vi "ex_GetAllExpressAttribsPlus.vi"(8 "error in":errorcluster, 11 "Signals in":waveform(dbl)[](array[waveform])) -> (0 "error out":errorcluster, 1 "All Express Wave Attributes Plus":T2(array[cluster]) {"dX" format="%.2f"; "X0" format="%<%X\n%x>T"; "Timestamp" format="%<%X\n%x>T"; "Start Timestamp" format="%<%X\n%x>T"}, 2 "All Express Wave Attributes":T1(array[cluster]) {"Timestamp" format="%<%X\n%x>T"; "Start Timestamp" format="%<%X\n%x>T"}, 3 "Signals out":waveform(dbl)[](array[waveform]), 5 "Time Attribs Not Found":bool[](array[boolean]))   [LabVIEW 2020]
doc: "Read Express attributes (and other Waveform values). If any of the four time-related attributes are not found, adds a best guess to the to All Express Wave Attributes."
uses:
  ex_WaveformAttribsPlus.ctl
  ex_WaveformAttribs.ctl
panel:
  in  "origin timestamps":timestamp[](array[timestamp]) format="%<%X\n%x>T"
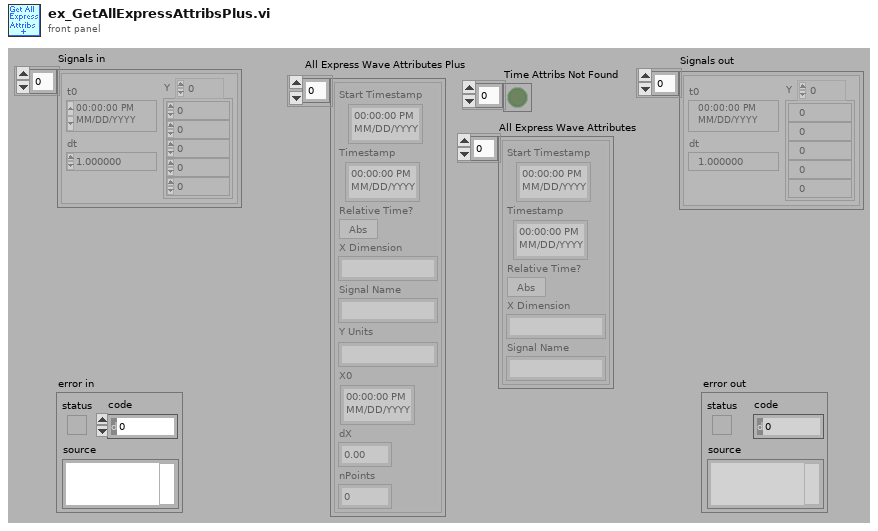
[diagram p1: front panel]
types:
  T1 = cluster{"Start Timestamp":timestamp, "Timestamp":timestamp, "Relative Time?":bool, "X Dimension":string, "Signal Name":string}[]
  T2 = cluster{"Start Timestamp":timestamp, "Timestamp":timestamp, "Relative Time?":bool, "X Dimension":string, "Signal Name":string, "Y Units":string, "X0":timestamp, "dX":dbl, "nPoints":i32}[]
  T3 = typedef "ex_WaveformAttribsPlus.ctl" = cluster{"Start Timestamp":timestamp, "Timestamp":timestamp, "Relative Time?":bool, "X Dimension":string, "Signal Name":string, "Y Units":string, "X0":timestamp, "dX":dbl, "nPoints":i32}
  T4 = typedef "ex_WaveformAttribs.ctl" = cluster{"Start Timestamp":timestamp, "Timestamp":timestamp, "Relative Time?":bool, "X Dimension":string, "Signal Name":string}
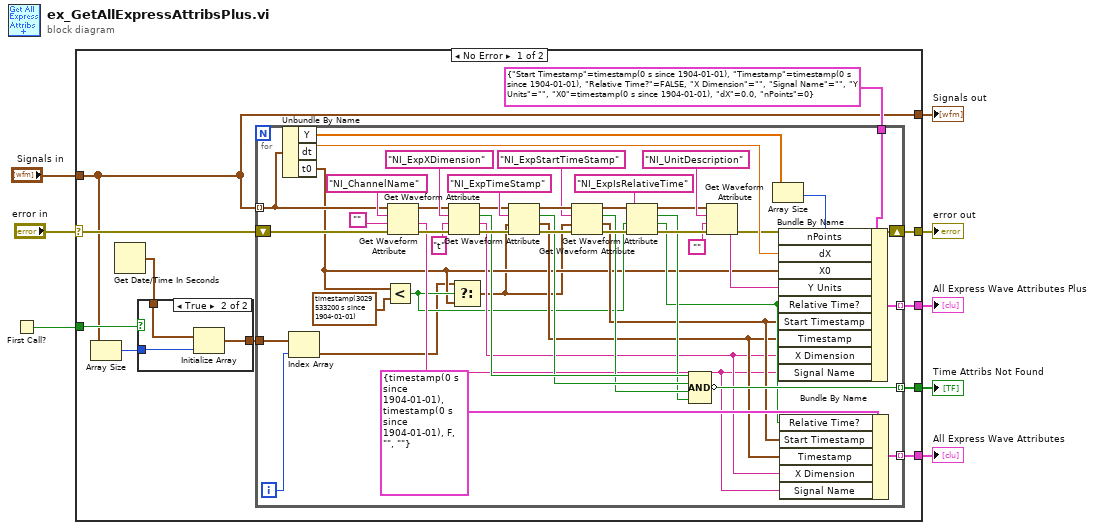
[diagram p0: block diagram]
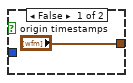
[diagram p2: hidden frame]
diagram:
  n1 = First Call?() -> (First Call?: T/F=w1:bool)
  n2 = case shown="No Error" "error in" {
    selector: "error in" -> [w19 w72]
    tunnel: [w15 w72] -> w8
    tunnel: "Signals in" -> [w11 w71]
    tunnel: [w16 _] -> w6
    tunnel: [w17 _] -> w4
    tunnel: [w11 w71] -> w3
    tunnel: [w14 _] -> w2
    tunnel: w1 -> [w12 _]
    frame No Error {
      n3 = Array Size(array=w11) -> (size(s)=w10:i32)
      n4 = Get Date/Time In Seconds() -> (seconds since 1Jan1904=w9:timestamp)
      n5 = case shown="True" w12 {
        tunnel: ["origin timestamps" w23] -> w13
        tunnel: w10 -> [_ w22]
        tunnel: w9 -> [_ w21]
        frame False {
        }
        frame True {
          n6 = Initialize Array(w21, w22) -> (w23:timestamp[])
        }
      }
      n7 = for {
        tunnel: w11 -> [w32] mode=indexing
        shift-right: [w47] -> w15
        shift-left: w19 -> [w62]
        tunnel: T3 {"Start Timestamp"=timestamp(0 s since 1904-01-01), "Timestamp"=timestamp(0 s since 1904-01-01), "Relative Time?"=FALSE, "X Dimension"="", "Signal Name"="", "Y Units"="", "X0"=timestamp(0 s since 1904-01-01), "dX"=0.0, "nPoints"=0} ("All Express Wave Attributes") -> [w56]
        tunnel: [w42] -> w17 mode=indexing
        tunnel: [w41] -> w16 mode=indexing
        tunnel: [w34] -> w14 mode=indexing
        tunnel: w13 -> [w28]
        i -> [w25]
        n8 = Unbundle By Name(w32) -> ("Y"=w50:dbl[], "dt"=w48:dbl, "t0"=w27:timestamp)
        n9 = Index Array(array=w28, index=w25) -> (element=w26:timestamp)
        n10 = Less?(x=w27, y=timestamp(3029533200 s since 1904-01-01) ("number")) -> (x < y?=w29:bool)
        n11 = Get Waveform Attribute(4:w62, 5:"", 6:"NI_ChannelName" ("name"), 7:w32) -> (0:w59:errorcluster, 1:w35:string, 3:w60:waveform(dbl))  [unwired: 1 out]
        n12 = Get Waveform Attribute(4:w59, 5:"t", 6:"NI_ExpXDimension" ("name"), 7:w60) -> (0:w57:errorcluster, 1:w36:string, 2:w46:bool, 3:w58:waveform(dbl))
        n13 = Select(t=w26, s=w29, f=w27) -> (s? t:f=w24:timestamp)
        n14 = Get Waveform Attribute(4:w57, 5:w24, 6:"NI_ExpTimeStamp" ("name"), 7:w58) -> (0:w66:errorcluster, 1:w37:timestamp, 2:w45:bool, 3:w67:waveform(dbl))
        n15 = Get Waveform Attribute(4:w66, 5:w24, 6:"NI_ExpStartTimeStamp" ("name"), 7:w67) -> (0:w69:errorcluster, 1:w38:timestamp, 2:w44:bool, 3:w70:waveform(dbl))
        n16 = Get Waveform Attribute(4:w69, 5:w29, 6:"NI_ExpIsRelativeTime" ("name"), 7:w70) -> (0:w53:errorcluster, 1:w39:bool, 2:w43:bool, 3:w54:waveform(dbl))
        n17 = Compound Arithmetic op=AND(w46, w45, w44, w43) -> (invert w42:bool)
        n18 = Get Waveform Attribute(4:w53, 5:"", 6:"NI_UnitDescription" ("name"), 7:w54) -> (0:w47:errorcluster, 1:w51:string)  [unwired: 2 out]
        n19 = Array Size(array=w50) -> (size(s)=w49:i32)
        n20 = Bundle By Name(cluster=w56, "nPoints"=w49, "dX"=w48, "X0"=w27, "Y Units"=w51, "Relative Time?"=w39, "Start Timestamp"=w38, "Timestamp"=w37, "X Dimension"=w36, "Signal Name"=w35) -> (w41:T3)
        n21 = Bundle By Name(cluster=T4 {"Start Timestamp"=timestamp(0 s since 1904-01-01), "Timestamp"=timestamp(0 s since 1904-01-01), "Relative Time?"=FALSE, "X Dimension"="", "Signal Name"=""} ("All Express Wave Attributes"), "Relative Time?"=w39, "Start Timestamp"=w38, "Timestamp"=w37, "X Dimension"=w36, "Signal Name"=w35) -> (w34:T4)
      }
    }
    frame Error {
    }
  }
  "error out" <- w8
  "All Express Wave Attributes Plus" <- w6
  "Time Attribs Not Found" <- w4
  "Signals out" <- w3
  "All Express Wave Attributes" <- w2
